vi "response.Has ID.vi"(8 "error in (no error)":errorcluster, 11 "Response in":refnum<class "Response.lvclass">) -> (0 "error out":errorcluster, 2 "has id?":bool, 3 "Response out":refnum<class "Response.lvclass">)   [LabVIEW 2020, in "JSON-RPC Lib.lvlib" / "Response.lvclass"]
uses:
  Response.lvclass
  Response.lvclass/Response.ctl
  id/id.Get ID Type.vi
  id/id.lvclass
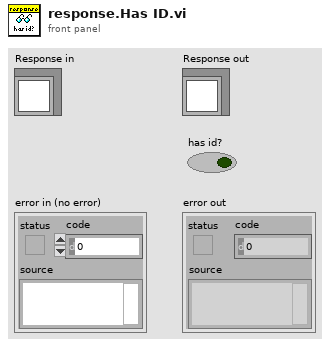
[diagram p1: front panel]
types:
  T1 = enum16{"String", "Numeric", "Boolean", "NULL", "Object", "Array"}
  T2 = typedef "NI_Data Type.lvlib/Data Type.ctl" = enum8{"Invalid Type", "Void", "I8", "I16", "I32", "I64", "U8", "U16", "U32", "U64", "Single Float", "Double Float", "Extended Float", "Single Complex", "Double Complex", "Extended Complex", "Enum U8", "Enum U16", "Enum U32", "Enum U64", "Single Float With Unit", "Double Float With Unit", "Extended Float With Unit", "Single Complex with Unit", "Double Complex with Unit", "Extended Complex with Unit", "Boolean", "String", "Path", "Picture", "Tag", "Array", "Cluster", "Variant", "LV Variant", "Waveform", "Timestamp", "Digital Waveform", "Digital Data", "ExpressData", "Refnum", "External Data", "VI", "Poly VI", "LabVIEW Class Instance", "Fixed Point", "Set Collection", "Map Collection"}
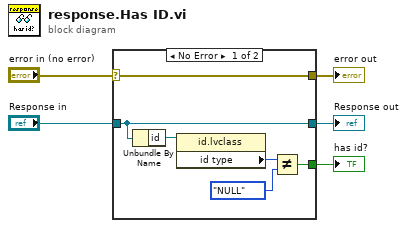
[diagram p0: block diagram]
diagram:
  n1 = case shown="No Error" "error in (no error)" {
    selector: "error in (no error)" -> [w11 w13]
    tunnel: [w11 w13] -> w4
    tunnel: [w10 w12] -> w2
    tunnel: "Response in" -> [w10 w12]
    tunnel: [w9 _] -> w1
    frame No Error {
      n2 = Unbundle By Name(w10) -> ("id"=w8:refnum<class "id.lvclass">)
      n3 = property class="id.lvclass"(reference=w8) -> ("id type"=w7:T2)  [unwired: 1 in, 2 out]
      n4 = Not Equal?(x=w7, y=T1."NULL") -> (x != y?=w9:bool)
    }
    frame Error {
    }
  }
  "error out" <- w4
  "Response out" <- w2
  "has id?" <- w1
